vi "Measurement UI.vi"() -> ()   [LabVIEW 2021, in "Single Tone_DAC_UI.lvlib"]
uses:
  Single Tone_DAC_UI.lvlib
  Single Tone_DAC.lvlib
panel:
  out "Freq domain":cluster{"x0":dbl, "dx":dbl, "magnitude":dbl[]}[](graph)
  out "Time domain graph":waveform(dbl)[](graph)
  out "Table results":string[][](table)
  in  "settings tab":enum32{"Measurement", "HiddenControls"}(tab)
  in  "Scope range (V)":dbl=5.0 caption="VERTICAL RANGE (V)" format="%.1p"
  in  "Scope samples":u32=50000 caption="NUMBER OF SAMPLES" format="%#.0p"
  in  "Scope channel":string="0" caption="CHANNEL"
  in  "Number of cycles":u32=200 caption="NUMBER OF CYCLES"
  in  "Number of bits":u32=16 caption="NUMBER OF BITS"
  in  "Amplitude stop (V)":dbl=4.93 caption="AMPLITUDE STOP (V)"
  in  "Full scale range (V)":dbl=5.0 caption="FULL SCALE RANGE (V)"
  in  "Scope sample rate (Hz)":dbl=50000.0 caption="SAMPLE RATE (Hz)" format="%#.0p"
  in  "Scope resource":string caption="SCOPE RESOURCE"
  in  "Amplitude start (V)":dbl=0.07 caption="AMPLITUDE START (V)"
  in  "Frequency (Hz)":dbl=1000.0 caption="FREQUENCY (Hz)" format="%#_6p"
  in  "DAC channel":u32 caption="DAC CHANNEL"
  in  "Digital resource":string caption="DIGITAL RESOURCE"
  out "ENOB":dbl[](array[numeric]) format="%_6g"
  out "THD (dB)":dbl[](array[numeric]) format="%_6g"
  out "SINAD (dB)":dbl[](array[numeric]) format="%_6g"
  out "SNR (dB)":dbl[](array[numeric]) format="%_6g"
  out "SFDR (dBc)":dbl[](array[numeric]) format="%_6g"
  out "Amplitude (dB)":dbl[](array[numeric]) format="%_6g"
  out "Amplitude (V)":dbl[](array[numeric]) format="%_6g"
  out "Frequency (Hz)":dbl[](array[numeric]) format="%_6g"
  out "df":dbl format="%_6g"
  out "f0":dbl format="%_6g"
  out "dt":dbl format="%_6g"
  out "Frequency domain":dbl[](array[numeric]) format="%_6g"
  out "Time domain":dbl[](array[numeric]) format="%_6g"
  out "Channel names":string[](array[string])
  # "Generation settings"
  # "Acquisition settings"
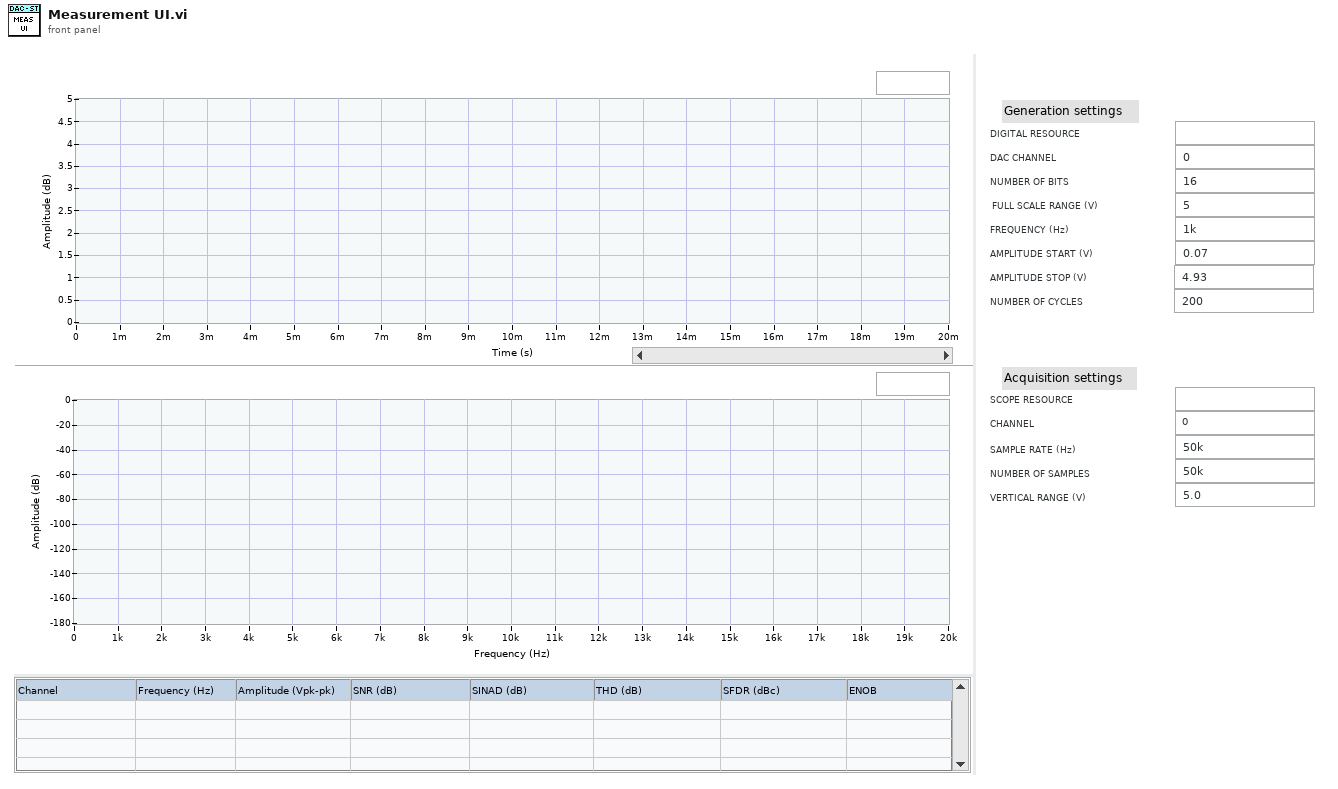
[diagram p1: front panel]
types:
  T1 = cluster{"Channel names":refnum<vi>, "Frequency":refnum<vi>, "Amplitude (V)":refnum<vi>, "SNR":refnum<vi>, "THD+N":refnum<vi>, "THD":refnum<vi>, "SFDR":refnum<vi>, "ENOB":refnum<vi>}
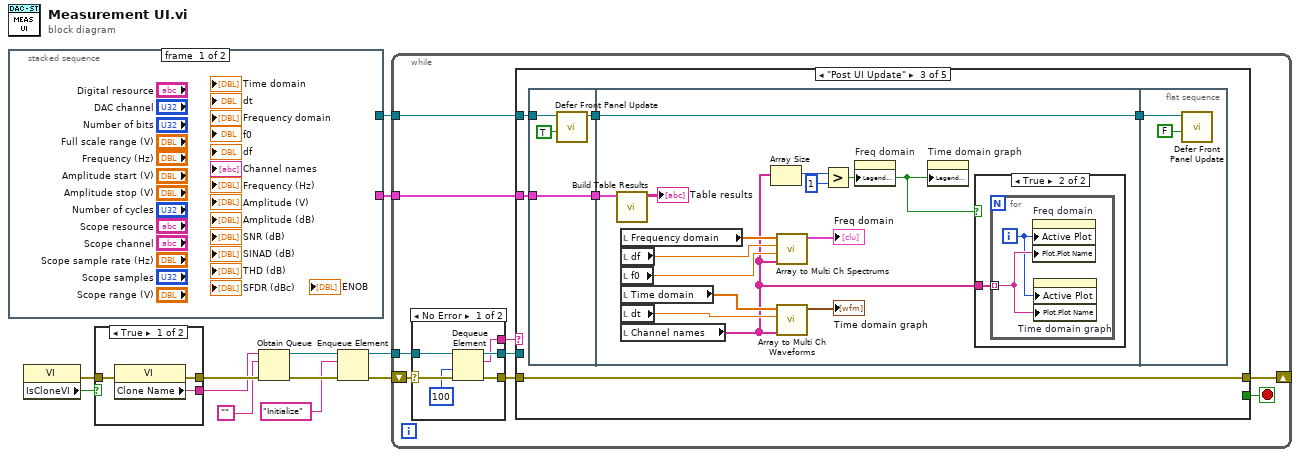
[diagram p0: block diagram]
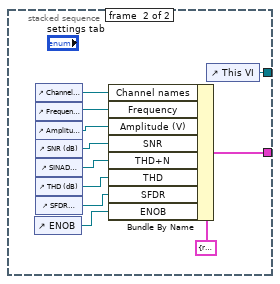
[diagram p2: hidden frame]
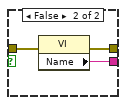
[diagram p3: hidden frame]
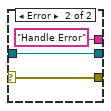
[diagram p4: hidden frame]
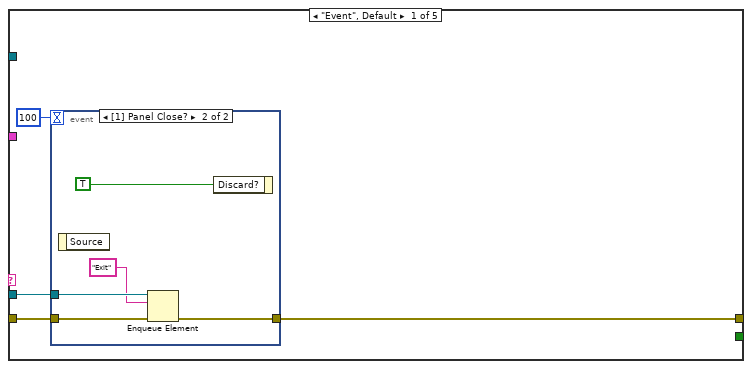
[diagram p5: hidden frame]
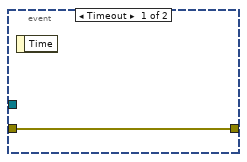
[diagram p6: hidden frame]
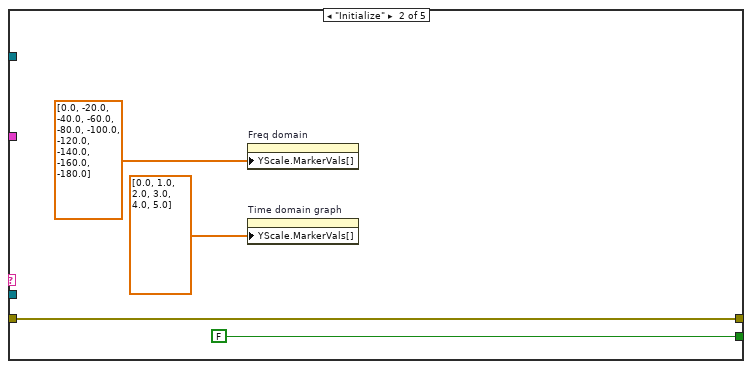
[diagram p7: hidden frame]
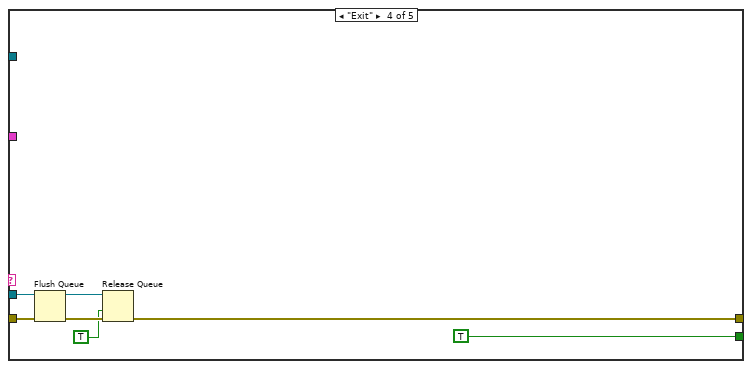
[diagram p9: hidden frame]
diagram:
  n1 = stacked-sequence {
    tunnel: [_ w15] -> w2
    tunnel: [_ w14] -> w1
    frame #0 {
    }
    frame #1 {
      n2 = control-ref of="ENOB"() -> (w13:refnum<vi>)
      n3 = control-ref of="Channel names"() -> (w22:refnum<vi>)
      n4 = control-ref of="Frequency (Hz)"() -> (w21:refnum<vi>)
      n5 = control-ref of="Amplitude (V)"() -> (w20:refnum<vi>)
      n6 = control-ref of="SNR (dB)"() -> (w19:refnum<vi>)
      n7 = control-ref of="SINAD (dB)"() -> (w18:refnum<vi>)
      n8 = control-ref of="THD (dB)"() -> (w17:refnum<vi>)
      n9 = control-ref of="SFDR (dBc)"() -> (w16:refnum<vi>)
      n10 = Bundle By Name(cluster=T1 {"Channel names"=refnum, "Frequency"=refnum, "Amplitude (V)"=refnum, "SNR"=refnum, "THD+N"=refnum, "THD"=refnum, "SFDR"=refnum, "ENOB"=refnum} ("Table result references"), "Channel names"=w22, "Frequency"=w21, "Amplitude (V)"=w20, "SNR"=w19, "THD+N"=w18, "THD"=w17, "SFDR"=w16, "ENOB"=w13) -> (w15:T1)
      n11 = control-ref of="This VI"() -> (w14:refnum<vi>)
    }
  }
  n12 = property class="VI"() -> (error out=w3:errorcluster, "IsCloneVI"=w4:bool)  [unwired: 2 in, 1 out]
  n13 = case shown="True" w4 {
    tunnel: [w26 w29] -> w12
    tunnel: [w25 w28] -> w11
    tunnel: w3 -> [w24 w27]
    frame True {
      n14 = property class="VI"(error in=w24) -> (error out=w26:errorcluster, "Clone Name"=w25:string)  [unwired: 1 in, 1 out]
    }
    frame False {
      n15 = property class="VI"(error in=w27) -> (error out=w29:errorcluster, "Name"=w28:string)  [unwired: 1 in, 1 out]
    }
  }
  n16 = Obtain Queue(name (unnamed)=w11, element data type="", error in (no error)=w12) -> (queue out=w8:refnum<queue>, error out=w10:errorcluster)  [unwired: 2 in, 1 out]
  n17 = Enqueue Element(queue=w8, element="Initialize", error in (no error)=w10) -> (queue out=w7:refnum<queue>, error out=w9:errorcluster)  [unwired: 1 in, 1 out]
  n18 = while {
    shift-right: [w33] -> _
    shift-left: w9 -> [w38]
    tunnel: w7 -> [w36]
    tunnel: w2 -> [w31]
    tunnel: w1 -> [w30]
    stop <- w32 stop-if-true
    n19 = case shown="No Error" w38 {
      selector: w38 -> [w44 w47]
      tunnel: [w43 w47] -> w37
      tunnel: w36 -> [w42 w46]
      tunnel: [w41 w46] -> w35
      tunnel: [w40 "Handle Error"] -> w34
      frame No Error {
        n20 = Dequeue Element(queue=w42, timeout in ms (-1)=100, error in (no error)=w44) -> (queue out=w41:refnum<queue>, element=w40:string, error out=w43:errorcluster)  [unwired: 1 out]
      }
      frame Error {
      }
    }
    n21 = case shown="\"Post UI Update\"" w34 {
      tunnel: w37 -> [w50 w61 w67 w97 w98]
      tunnel: w35 -> [w48 _ _ w95 _]
      tunnel: [w51 w61 w67 w92 w98] -> w33
      tunnel: [_ FALSE _ TRUE _] -> w32
      tunnel: w31 -> [_ _ w66 _ _]
      tunnel: w30 -> [_ _ w64 _ _]
      frame "Event", Default {
        n22 = event shown="[1] Panel Close?" {
          selector: _ -> [_ _]
          dyn-events: _ -> [_ _]
          timeout: 100 -> [_ _]
          tunnel: [w52 w55] -> w51
          tunnel: w50 -> [w52 w56]
          tunnel: w48 -> [_ w54]
          event Timeout {
            n23 = event-data() -> ()  [unwired: 1 in, 1 out]
          }
          event Panel Close? {
            n24 = event-data() -> ()  [unwired: 1 in, 1 out]
            n25 = Enqueue Element(queue=w54, element="Exit", error in (no error)=w56) -> (error out=w55:errorcluster)  [unwired: 1 in, 2 out]
            n26 = event-data("Discard?"=TRUE) -> ()  [unwired: 1 in, 1 out]
          }
        }
      }
      frame "Initialize" {
        n27 = property on="Freq domain" class="WFGraph (strict)"("YScale.MarkerVals[]"=dbl[] [0.0, -20.0, -40.0, -60.0, -80.0, -100.0, -120.0, -140.0, -160.0, -180.0] ("Y Scale.Marker Values[]")) -> ()  [unwired: 2 in, 2 out]
        n28 = property on="Time domain graph" class="WFGraph (strict)"("YScale.MarkerVals[]"=dbl[] [0.0, 1.0, 2.0, 3.0, 4.0, 5.0] ("Y Scale.Marker Values[]")) -> ()  [unwired: 2 in, 2 out]
      }
      frame "Post UI Update" {
        # "This case will be triggered, after framework updates the User interface with result values."
        n29 = flat-sequence {
          tunnel: w66 -> [w71]
          tunnel: [w71] -> w65
          tunnel: w64 -> [w70]
          tunnel: [w68] -> w63
          tunnel: w65 -> [w77]
          tunnel: w63 -> [w72]
          tunnel: [w72] -> w62
          tunnel: w62 -> [w90]
          frame #0 {
            n30 = call "Defer Front Panel Update.vi"("Defer Panel Updates"=TRUE, "VI in"=w70) -> ("VI out"=w68:refnum<vi>)  [unwired: 8 in, 1 out]
          }
          frame #1 {
            n31 = call "Build Table Results.vi"("Table result references"=w77) -> ("Table values"=→"Table results":string[][])  [unwired: 10 in]
            n32 = local read "Frequency domain"() -> (w82:dbl[])
            n33 = local read "df"() -> (w81:dbl)
            n34 = local read "f0"() -> (w80:dbl)
            n35 = local read "Time domain"() -> (w85:dbl[])
            n36 = local read "dt"() -> (w84:dbl)
            n37 = local read "Channel names"() -> (w74:string[])
            n38 = Array Size(array=w74) -> (size(s)=w76:i32)
            n39 = call "Array to Multi Ch Spectrums.vi"("channel names"=w74, "f0"=w80, "df"=w81, "array"=w82) -> ("spectra"=→"Freq domain":cluster{"x0":dbl, "dx":dbl, "magnitude":dbl[]}[])  [unwired: 7 in]
            n40 = call "Array to Multi Ch Waveforms.vi"("channel names"=w74, "dt"=w84, "array"=w85) -> ("waveforms"=→"Time domain graph":waveform(dbl)[])  [unwired: 8 in]
            n41 = Greater?(x=w76, y=1) -> (0:w73:bool)
            n42 = property on="Freq domain" class="WFGraph (strict)"("Legend Visible"=w73) -> ()  [unwired: 2 in, 2 out]
            n43 = property on="Time domain graph" class="WFGraph (strict)"("Legend Visible"=w73) -> ()  [unwired: 2 in, 2 out]
            n44 = case shown="True" w73 {
              tunnel: w74 -> [_ w86]
              frame False {
              }
              frame True {
                n45 = for {
                  tunnel: w86 -> [w88] mode=indexing
                  i -> [w87]
                  n46 = property on="Freq domain" class="WFGraph (strict)"("Active Plot"=w87, "Plot.Plot Name"=w88) -> ()  [unwired: 2 in, 2 out]
                  n47 = property on="Time domain graph" class="WFGraph (strict)"("Active Plot"=w87, "Plot.Plot Name"=w88) -> ()  [unwired: 2 in, 2 out]
                }
              }
            }
          }
          frame #2 {
            n48 = call "Defer Front Panel Update.vi"("Defer Panel Updates"=FALSE, "VI in"=w90) -> ()  [unwired: 8 in, 2 out]
          }
        }
      }
      frame "Exit" {
        # "This case is triggered to close the User Interface from framework"
        n49 = Flush Queue(queue=w95, error in (no error)=w97) -> (queue out=w94:refnum<queue>, error out=w93:errorcluster)  [unwired: 1 out]
        n50 = Release Queue(queue=w94, force destroy? (F)=TRUE, error in (no error)=w93) -> (error out=w92:errorcluster)  [unwired: 2 out]
      }
      frame "Handle Error" {
      }
    }
  }
